vi "Query with 2D String Result.vi"(8 "error in (no error)":errorcluster, 10 "Query string":string, 11 "sqlite3 in":refnum<class "sqlite3.lvclass">) -> (0 "error out":errorcluster, 2 "Result":string[][](array[string]), 3 "sqlite3 out":refnum<class "sqlite3.lvclass">)   [LabVIEW 2020, in "sqlite3.lvlib" / "sqlite3.lvclass"]
uses:
  sqlite3.lvclass
  sqlite3.lvclass/sqlite3.ctl
  e4de3e57-8ce3-4d5b-8aad-e4f289183583.vi
  sqlite/VIs/open v2.vi
  sqlite/VIs/close v2.vi
  sqlite/VIs/prepare v2.vi
  sqlite/VIs/step.vi
  sqlite/VIs/column count.vi
  db layer/compound/Resolve Result Type.vi
  e4de3e57-8ce3-4d5b-8aad-e4f289183583.vi/7bc19fd7-2686-4951-aa35-a0d62870a61f.vi
  e4de3e57-8ce3-4d5b-8aad-e4f289183583.vi/0c990a8c-7110-4797-b890-0104de729f69.vi
  sqlite/VIs/finalize.vi
  sqlite/subvi/Error Converter (ErrCode or Status).vi
  sqlite/VIs/column type.vi
  sqlite/VIs/column text.vi
  sqlite/VIs/column bytes.vi
  sqlite/VIs/column blob.vi
  db layer/utilities/MoveBlock.vi
  sqlite/VIs/errstr.vi
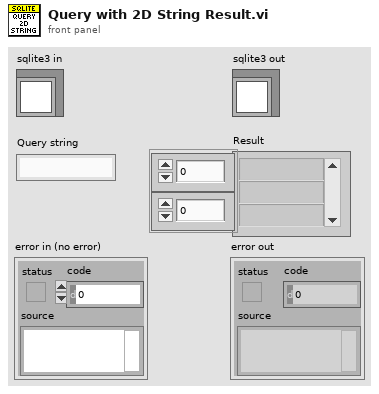
[diagram p1: front panel]
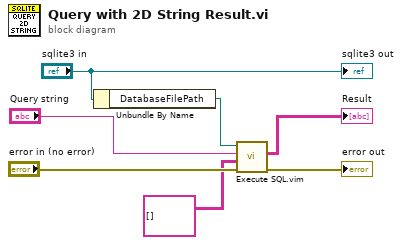
[diagram p0: block diagram]
diagram:
  n1 = Unbundle By Name("sqlite3 in") -> ("DatabaseFilePath"=w1:path)
  n2 = call "Execute SQL.vim"("error in (no error)"="error in (no error)", "desired return type(none)"=string[][] [] ("Result"), "sql (string)"="Query string", "database in"=w1) -> ("error out"=→"error out":errorcluster, "Query Result"=→"Result":string[][])  [unwired: 6 in]
  "sqlite3 out" <- "sqlite3 in"
